vi "HSDIO_6541_Init_Session.vi"(8 "error in (no error)":errorcluster, 10 "Use Software Trigger":bool=TRUE, 11 "HSDIO 6541 Inputs":T1={"Resource Name"="HSDIO_6541", "Clock Rate"=1000000.0, "Trigger Source"="PFI0"} {"Clock Rate" format="%.2p"}) -> (0 "error out":errorcluster, 3 "instrument handle out":refnum<k15>)   [LabVIEW 2024]
doc: "This VI inits a waveform generation session for HSDIO 6541. This is a basic example that shows how to setup the board in order to generate waveforms according to a script. \n\n1. Initialize for a generation session.\n2. Assign specified channels in Channel List for dynamic operation : all = \"\" (default)\n3. Sets the Idle State when the generation has completed : NO !!\n4. Configure the Sample clock to use (onboard clock), and configure the clock rate.\n5. Set generation mode to Scripted.\n6. Configure the Script Trigger : change to Digital Edge if waiting for an external\n trigger, and link Rising Edge and source trigger commands.\n Use PFI0 with SMB wired to the board, or any PFIxx if connected to accessory."
uses:
  controls/HSDIO_6541_Inputs.ctl
  <instrlib>/niHSDIO/niHSDIO.llb/niHSDIO_ctl Trigger Source Values (Ring).ctl
  <instrlib>/niHSDIO/niHSDIO.llb/niHSDIO_ctl Generation Mode Values (Ring).ctl
  <instrlib>/niHSDIO/niHSDIO.llb/niHSDIO_ctl Sample Clock Source Values (ComboBox).ctl
  <instrlib>/niHSDIO/niHSDIO.llb/niHSDIO_ctl Trigger DigEdge - Edge Values (Ring).ctl
  <instrlib>/niHSDIO/niHSDIO.llb/niHSDIO_ctl Trigger Script - trigID Values (Ring).ctl
  <instrlib>/niHSDIO/niHSDIO.llb/niHSDIO Configure Digital Edge Script Trigger.vi
  <instrlib>/niHSDIO/niHSDIO.llb/niHSDIO Configure Software Script Trigger.vi
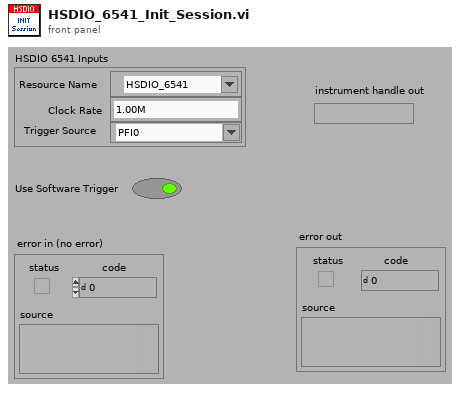
[diagram p1: front panel]
types:
  T1 = typedef "HSDIO_6541_Inputs.ctl" = cluster{"Resource Name":refnum<k15>, "Clock Rate":dbl, "Trigger Source":T2}
  T2 = typedef "niHSDIO_ctl Trigger Source Values (Ring).ctl" = string
  T3 = typedef "niHSDIO_ctl Sample Clock Source Values (ComboBox).ctl" = string
  T4 = typedef "niHSDIO_ctl Trigger Script - trigID Values (Ring).ctl" = string
  T5 = typedef "niHSDIO_ctl Generation Mode Values (Ring).ctl" = i32
  T6 = typedef "niHSDIO_ctl Trigger DigEdge - Edge Values (Ring).ctl" = i32
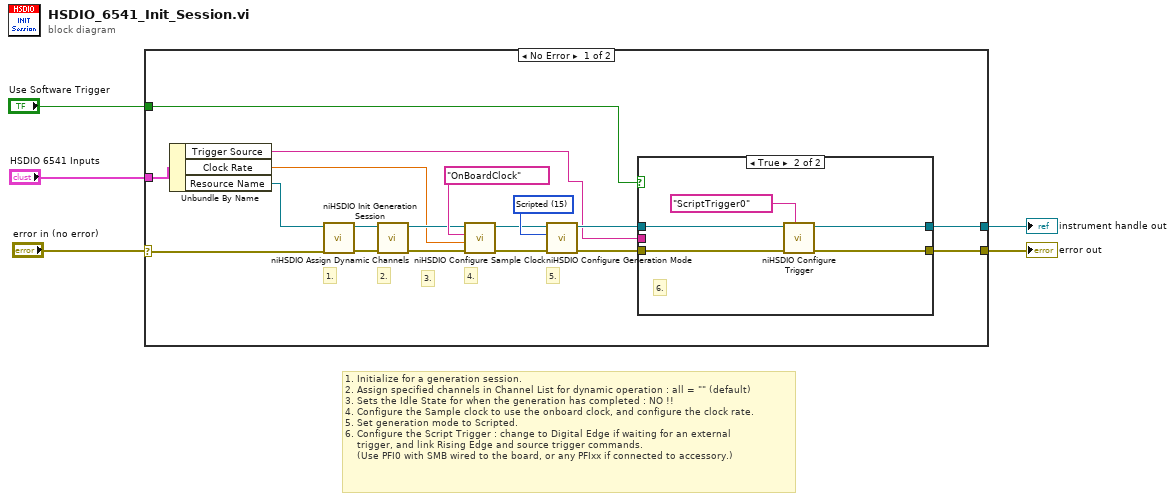
[diagram p0: block diagram]
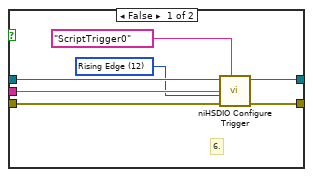
[diagram p2: hidden frame]
diagram:
  # "1. Initialize for a generation session.\n2. Assign specified channels in Channel List for dynamic operation : all = \"\" (default)\n3. Sets the Idle State for when the generation has completed : NO !!\n4. Configure the Sample clock to use the onboard clock, and configure the clock rate.\n5. Set generation mode to Scripted.\n6. Configure the Script Trigger : change to Digital Edge if waiting for an external\n    trigger, and link Rising Edge and source trigger commands.\n    (Use PFI0 with SMB wired to the board, or any PFIxx if connected to accessory.)"
  n1 = case shown="No Error" "error in (no error)" {
    selector: "error in (no error)" -> [w6 w36]
    tunnel: [w23 _] -> w5
    tunnel: [w22 w36] -> w4
    tunnel: "Use Software Trigger" -> [w21 _]
    tunnel: "HSDIO 6541 Inputs" -> [w7 _]
    frame No Error {
      w17 = T5 15 items=["Waveform"=14, "Scripted"=15] ("generation mode (waveform)")
      # "5."
      # "4."
      # "3."
      # "2."
      # "1."
      n2 = Unbundle By Name(w7) -> ("Trigger Source"=w9:T2, "Clock Rate"=w10:dbl, "Resource Name"=w8:refnum<k15>)
      n3 = call <instrlib>:"niHSDIO Init Generation Session.vi"("error in (no error)"=w6, "resource name"=w8) -> ("error out"=w19:errorcluster, "instrument handle out"=w20:refnum<k15>)  [unwired: 8 in]
      n4 = call <instrlib>:"niHSDIO Assign Dynamic Channels.vi"("error in (no error)"=w19, "instrument handle"=w20) -> ("error out"=w13:errorcluster, "instrument handle out"=w14:refnum<k15>)  [unwired: 8 in]
      n5 = call <instrlib>:"niHSDIO Configure Sample Clock.vi"("error in (no error)"=w13, "clock rate (50MHz)"=w10, "clock source (on board clock)"=T3 "OnBoardClock", "instrument handle"=w14) -> ("error out"=w15:errorcluster, "instrument handle out"=w16:refnum<k15>)  [unwired: 6 in]
      n6 = call <instrlib>:"niHSDIO Configure Generation Mode.vi"("error in (no error)"=w15, "generation mode (waveform)"=w17, "instrument handle"=w16) -> ("error out"=w11:errorcluster, "instrument handle out"=w12:refnum<k15>)  [unwired: 7 in]
      n7 = case shown="True" w21 {
        tunnel: w12 -> [w30 w35]
        tunnel: w11 -> [w29 w34]
        tunnel: [w28 w33] -> w23
        tunnel: [w27 w32] -> w22
        tunnel: w9 -> [w26 _]
        frame False {
          w25 = T6 12 items=["Rising Edge"=12, "Falling Edge"=13] ("Edge")
          # "6."
          n8 = call-poly <instrlib>:"niHSDIO Configure Trigger.vi"("trigger id (script trigger 0)"=T4 "ScriptTrigger0", "error in (no error)"=w29, "edge (rising)"=w25, "source (PFI 0)"=w26, "instrument handle"=w30) -> ("error out"=w27:errorcluster, "instrument handle out"=w28:refnum<k15>)  [unwired: 5 in]
        }
        frame True {
          # "6."
          n9 = call-poly <instrlib>:"niHSDIO Configure Trigger.vi"("trigger id (script trigger 0)"=T4 "ScriptTrigger0", "error in (no error)"=w34, "instrument handle"=w35) -> ("error out"=w32:errorcluster, "instrument handle out"=w33:refnum<k15>)  [unwired: 7 in]
        }
      }
    }
    frame Error {
    }
  }
  "instrument handle out" <- w5
  "error out" <- w4
